vi "main_v2.vi"() -> ()   [LabVIEW 2017]
uses:
  <vilib>/DAQmx/read.llb/DAQmx Read (Analog 2D DBL NChan NSamp).vi
  <vilib>/DAQmx/configure/timing.llb/DAQmx Timing (Sample Clock).vi
  <vilib>/DAQmx/miscellaneous.llb/DAQmx Fill In Error Info.vi
panel:
  in  "Scale b":dbl[](array[numeric])
  in  "Scale a":dbl[](array[numeric])
  out "drehmoment_kraft":dbl[][](graph)
  out "temperature":dbl[][](graph)
  in  "stop":bool
  # "y = a * x + b"
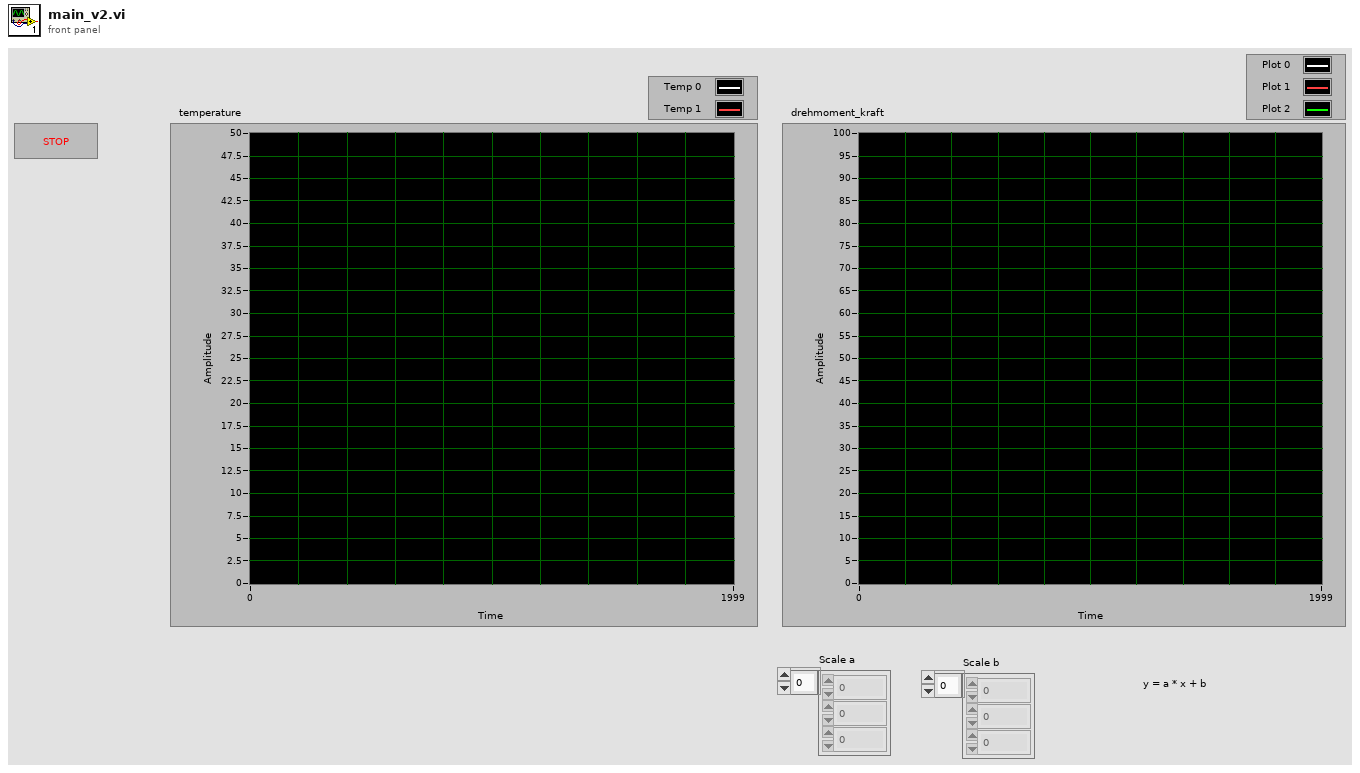
[diagram p1: front panel]
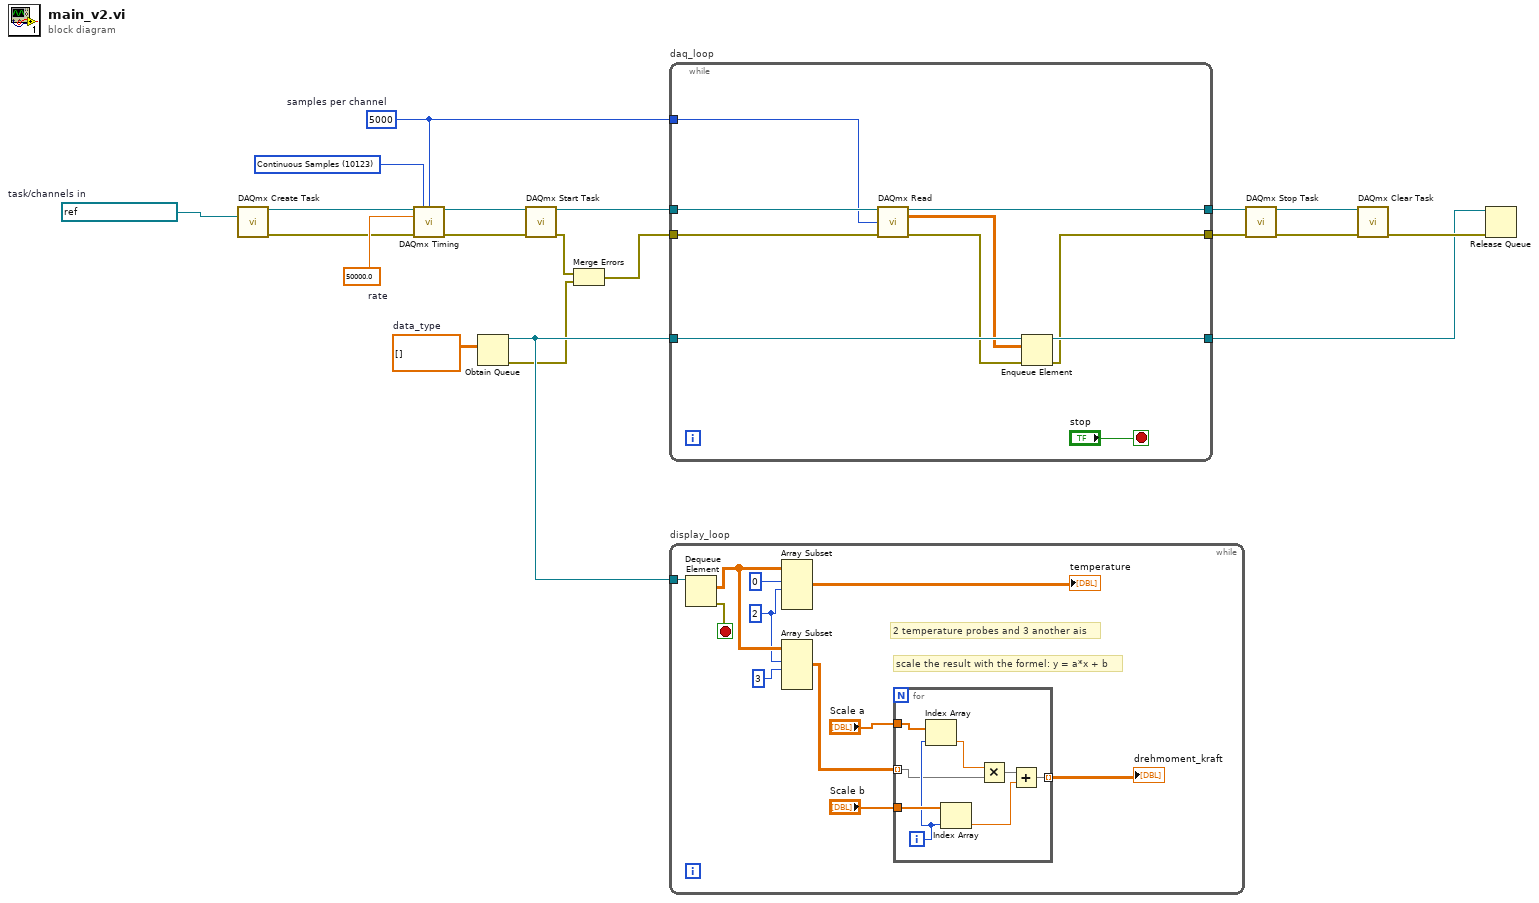
[diagram p0: block diagram]
diagram:
  w14 = dbl[][] []  # data_type
  w19 = 50000.0  # rate
  w1 = 5000  # samples per channel
  w20 = 10123 items=["Finite Samples"=10178, "Continuous Samples"=10123, "Hardware Timed Single Point"=12522] ("sample mode")
  w6 = refnum<k21> "AnalogReadTask"  # task/channels in
  n1 = call <vilib>:"DAQmx Create Task.vi"("task to copy"=w6) -> ("task out"=w7:refnum<k21>, "error out"=w8:errorcluster)  [unwired: 13 in]
  n2 = call-poly <vilib>:"DAQmx Timing.vi"("task/channels in"=w7, "sample mode"=w20, "samples per channel"=w1, "rate"=w19, "error in"=w8) -> ("task out"=w3:refnum<k21>, "error out"=w2:errorcluster)  [unwired: 9 in]
  n3 = Obtain Queue(element data type=w14) -> (queue out=w13:refnum<queue>, error out=w10:errorcluster)  [unwired: 4 in, 1 out]
  n4 = call <vilib>:"DAQmx Start Task.vi"("task/channels in"=w3, "error in"=w2) -> ("task out"=w5:refnum<k21>, "error out"=w4:errorcluster)  [unwired: 12 in]
  n5 = Merge Errors(w4, w10) -> (w15:errorcluster)
  n6 = while "daq_loop" {
    tunnel: w15 -> [w29]
    tunnel: w5 -> [w28]
    tunnel: [w27] -> w18
    tunnel: w13 -> [w26]
    tunnel: [w25] -> w11
    tunnel: [w23] -> w9
    tunnel: w1 -> [w21]
    stop <- "stop" stop-if-true
    n7 = call-poly <vilib>:"DAQmx Read.vi"("task/channels in"=w28, "number of samples per channel"=w21, "error in"=w29) -> ("task out"=w27:refnum<k21>, "data"=w22:dbl[][], "error out"=w24:errorcluster)  [unwired: 10 in]
    n8 = Enqueue Element(queue=w26, element=w22, error in (no error)=w24) -> (queue out=w25:refnum<queue>, error out=w23:errorcluster)  [unwired: 1 in, 1 out]
  }
  n9 = while "display_loop" {
    tunnel: w13 -> [w41]
    stop <- w40 stop-if-true
    w33 = 2 ("length")
    # "2 temperature probes and 3 another ais"
    # "scale the result with the formel: y = a*x + b"
    n10 = Dequeue Element(queue=w41) -> (element=w36:dbl[][], error out=w40:errorcluster)  [unwired: 2 in, 2 out]
    n11 = Array Subset(array=w36, index (row)=0 ("index"), length (row)=w33) -> (→"temperature":dbl[][])  [unwired: 2 in]
    n12 = Array Subset(array=w36, index (row)=w33, length (row)=3 ("length")) -> (w34:dbl[][])  [unwired: 2 in]
    n13 = for {
      tunnel: "Scale a" -> [w46]
      tunnel: "Scale b" -> [w45]
      tunnel: [w48] -> w32 mode=indexing
      tunnel: w34 -> [w42] mode=indexing
      i -> [w44]
      n14 = Index Array(array=w46, index=w44) -> (element=w47:dbl)
      n15 = Index Array(array=w45, index=w44) -> (element=w43:dbl)
      n16 = Multiply(x=w47, y=w42) -> (x*y=w49:dbl[])
      n17 = Add(x=w49, y=w43) -> (x+y=w48:dbl[])
    }
    "drehmoment_kraft" <- w32
  }
  n18 = call <vilib>:"DAQmx Stop Task.vi"("task/channels in"=w18, "error in"=w9) -> ("task out"=w16:refnum<k21>, "error out"=w17:errorcluster)  [unwired: 12 in]
  n19 = call <vilib>:"DAQmx Clear Task.vi"("task in"=w16, "error in"=w17) -> ("error out"=w12:errorcluster)  [unwired: 13 in]
  n20 = Release Queue(queue=w11, error in (no error)=w12) -> ()  [unwired: 1 in, 3 out]
